vi "Write IndexInList.vi"(8 "error in (no error)":errorcluster, 10 "TestNum":u32, 11 "TestMeasureStep in":refnum<class "TestMeasureStep.lvclass">) -> (0 "error out":errorcluster, 3 "TestMeasureStep out":refnum<class "TestMeasureStep.lvclass">)   [LabVIEW 2017, in "TestMeasureStep.lvclass"]
uses:
  TestMeasureStep.lvclass
  TestMeasureStep.lvclass/TestMeasureStep.ctl
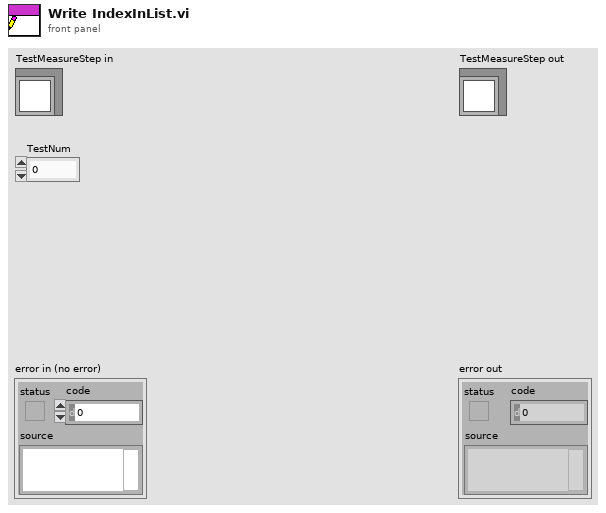
[diagram p1: front panel]
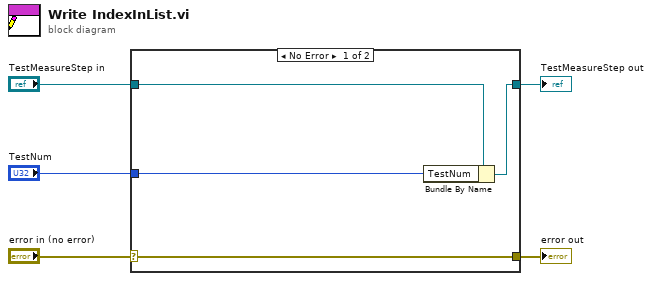
[diagram p0: block diagram]
diagram:
  n1 = case shown="No Error" "error in (no error)" {
    selector: "error in (no error)" -> [w9 w10]
    tunnel: [w9 w10] -> w4
    tunnel: [w7 w11] -> w2
    tunnel: "TestMeasureStep in" -> [w8 w11]
    tunnel: "TestNum" -> [w6 _]
    frame No Error {
      n2 = Bundle By Name(cluster=w8, "TestNum"=w6) -> (w7:refnum<class "TestMeasureStep.lvclass">)
    }
    frame Error {
    }
  }
  "error out" <- w4
  "TestMeasureStep out" <- w2
